vi "Exp03_GetGyroAngle.vi"() -> ()   [LabVIEW 2019]
uses:
  <vilib>/myRIO/Instrument Drivers/Onboard IO/I2C/typedefs/I2C User Configuration.ctl
  <vilib>/myRIO/Instrument Drivers/Onboard IO/I2C/typedefs/I2C Transfer Rate.ctl
  <vilib>/Platform/TimedLoop/XDataNode/timing_clust.ctl
  <vilib>/Platform/TimedLoop/XDataNode/nitl_modes.ctl
  <vilib>/Platform/TimedLoop/XDataNode/wakeup.ctl
  <vilib>/Utility/error.llb/Error Cluster From Error Code.vi
  <vilib>/myRIO/Common/Instrument Driver Framework/myRIO v1.0/I2C/vis/myRIO v1.0 Configure I2C.vi
  <vilib>/myRIO/Common/Instrument Driver Framework/myRIO v1.0/I2C/vis/myRIO v1.0 Write I2C.vi
  <vilib>/myRIO/Common/Instrument Driver Framework/myRIO v1.0/I2C/vis/myRIO v1.0 Read I2C.vi
  <vilib>/Platform/TimedLoop/XDataNode/XDataNode.xnode
  <vilib>/myRIO/Instrument Drivers/Onboard IO/I2C/I2C.lvlib
  <vilib>/Platform/TimedLoop/XDataNode/XDNodeRunTimeDep.lvlib
panel:
  out "gyro angle":dbl
  in  "zero":bool
  in  "initial bias":i16
  out "angular velocity":dbl
  out "acc angle":dbl
  out "Bytes Read (decimal)":u8[](array[numeric]) format="%0d"
  out "Gyro Z":i16
  out "Gyro X":i16
  out "Gyro Y":i16
  out "Acc Z":i16
  out "Temperature":dbl
  out "Acc Y":i16
  out "Acc X":i16
  in  "stop":bool
  out "error out":errorcluster
  out "Bytes Read (binary)":u8[](array[numeric]) format="%08b"
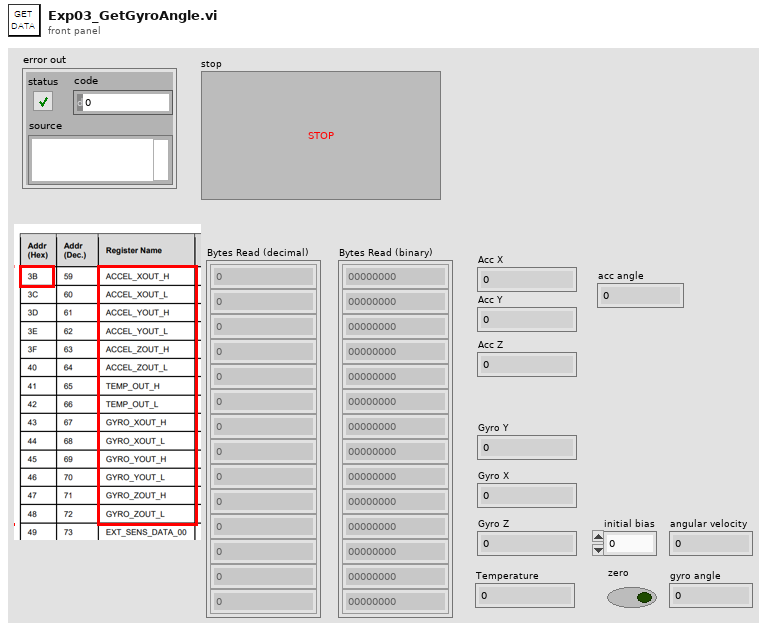
[diagram p1: front panel]
types:
  T1 = typedef "I2C.lvlib/I2C User Configuration.ctl" = cluster{"I2C Transfer Rate":T2}
  T2 = typedef "I2C.lvlib/I2C Transfer Rate.ctl" = enum16{"Standard mode (100 kbps)", "Fast mode (400 kbps)"}
  T3 = typedef "I2C.lvlib/I2C Reference.ctl" = cluster{"myRIO Reference":T4, "I2C Channels Enum":T8, "I2C Configuration":T9}
  T4 = typedef "myRIO Generic Hardware Reference.ctl" = cluster{"myRIO Model":T5, "myRIO Hardware Reference":T6}
  T5 = typedef "Hardware Version Enum.ctl" = enum16{"Unknown", "myRIO-1900", "myRIO-1950", "roboRIO", "NI ELVIS RIO CM", "ELVIS III"}
  T6 = typedef "myRIO v1.0 Reference.ctl" = cluster{"Generic FPGA Reference":T7, "Allow multiple opens":bool}
  T7 = typedef "Generic FPGA Reference.ctl" = refnum<k20>
  T8 = typedef "I2C Channels Enum.ctl" = enum16{"Not Connected", "A/I2C", "B/I2C", "I2C/I2C"}
  T9 = typedef "I2C.lvlib/I2C Configuration.ctl" = cluster{"I2C Transfer Rate":T2}
  T10 = typedef "XDNodeRunTimeDep.lvlib/timing_clust.ctl" = cluster{"Expected End [f-1]":u64, "Actual End [f-1]":u64, "Finished Late? [f-1]":bool, "Expected End [i-1]":u64, "Actual End [i-1]":u64, "Finished Late? [i-1]":bool, "Expected Start [i]":u64, "Actual Start [i]":u64, "Expected Start [f]":u64, "Actual Start [f]":u64, "Source Name":string, "Structure Name":string, "Period":i64, "Deadline":i64, "Offset":i64, "Start":i64, "Priority":i32, "Timeout":i32, "Mode":T11, "Wakeup Reason":T12, "Error":errorcluster, "Source Type":string, "Secondary Source Type":string, "Global End Time":u64, "Global Start Time":u64, "Frame Duration":u64, "Iteration Duration":u64, "Assigned CPU":i32, "I/O Scan Engine Mode":u32}
  T11 = typedef "XDNodeRunTimeDep.lvlib/nitl_modes.ctl" = enum32{"No Change", "Process missed periods, maintain original phase", "Discard missed periods, maintain original phase", "Process missed periods, ignore original phase", "Discard missed periods, ignore original phase"}
  T12 = typedef "XDNodeRunTimeDep.lvlib/wakeup.ctl" = enum32{"Normal", "Aborted", "Asynchronous wakeup", "Timing source error", "Timed loop error", "Timeout"}
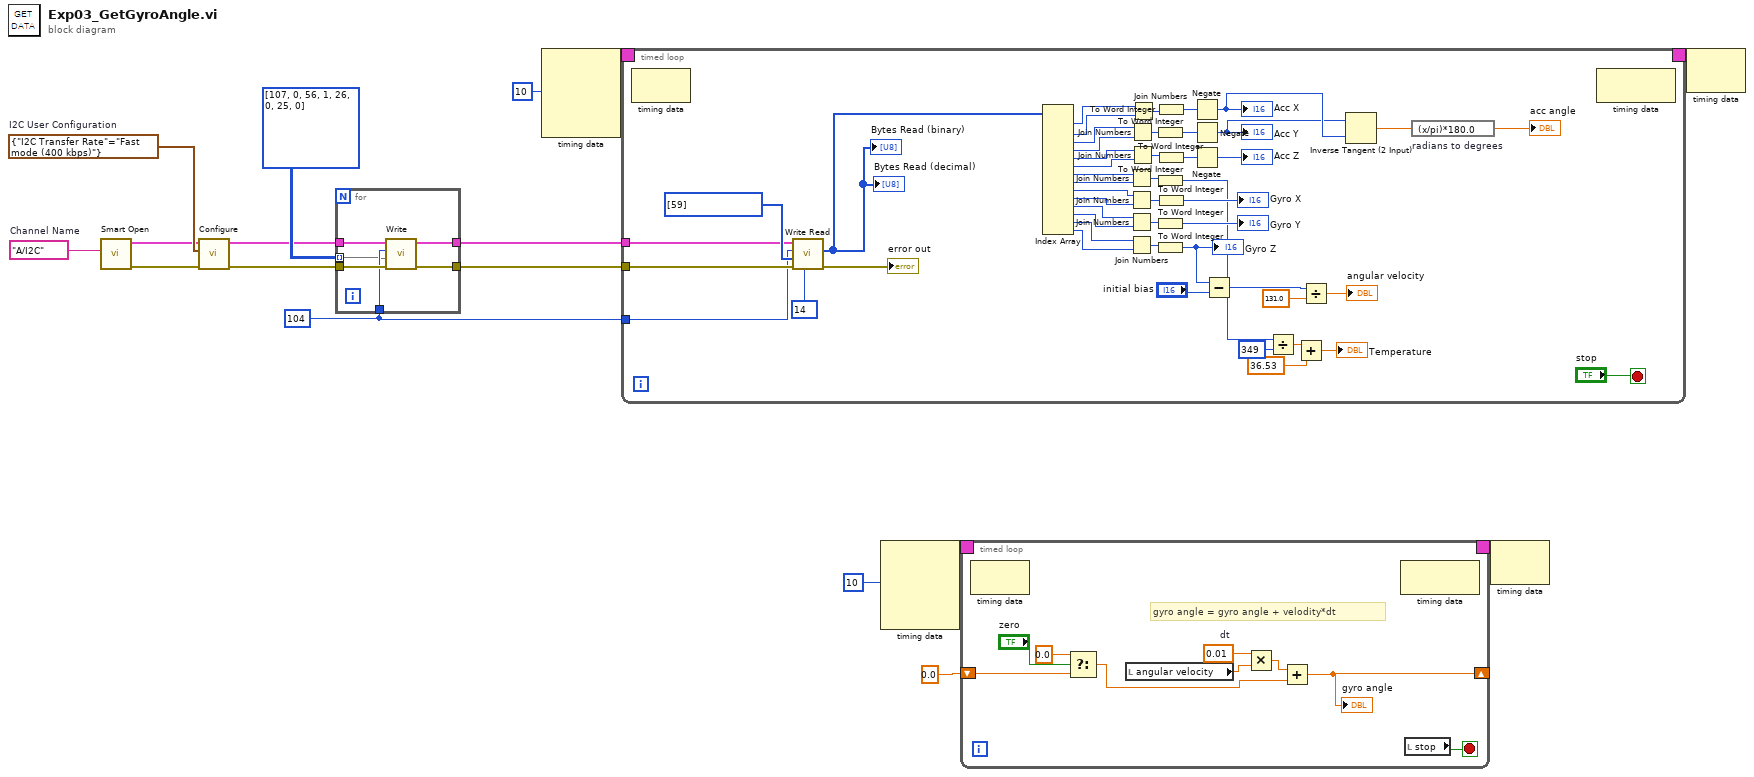
[diagram p0: block diagram]
diagram:
  w11 = u8 104 ("Slave Address (7-bit)")
  w16 = T1 {"I2C Transfer Rate"=enum."Fast mode (400 kbps)"}  # I2C User Configuration
  w17 = tag "A/I2C"  # Channel Name
  n1 = call <vilib>:"Smart Open.vi"("Channel Name"=w17) -> ("error out"=w14:errorcluster, "I2C Ref Out"=w15:T3)  [unwired: 9 in]
  n2 = call <vilib>:"Configure.vi"("error in (no error)"=w14, "I2C User Configuration"=w16, "I2C Ref In"=w15) -> ("error out"=w5:errorcluster, "I2C Ref Out"=w6:T3)  [unwired: 7 in]
  n3 = for {
    tunnel: w11 -> [w19]
    tunnel: w6 -> [w23]
    tunnel: [w20] -> w12
    tunnel: w5 -> [w22]
    tunnel: [w21] -> w13
    tunnel: u8[][] [[107, 0], [56, 1], [26, 0], [25, 0]] ("Bytes to Write") -> [w18] mode=indexing
    n4 = call <vilib>:"Write.vi"("error in (no error)"=w22, "Bytes to Write"=w18, "Slave Address (7-bit)"=w19, "I2C Ref In"=w23) -> ("error out"=w21:errorcluster, "I2C Ref Out"=w20:T3)  [unwired: 6 in]
  }
  n5 = node-c288(i64 10 ("Period")) -> (w10:T10)  [unwired: 3 in]
  n6 = timed-loop {
    timing: w10 -> [_]
    timing-out: [_] -> w9
    tunnel: w13 -> [w69]
    tunnel: w12 -> [w68]
    tunnel: w11 -> [w67]
    stop <- "stop" stop-if-true
    n7 = node-c288() -> ()  [unwired: 1 in, 1 out]
    n8 = call <vilib>:"Write Read.vi"("Byte Count"=u32 14, "error in (no error)"=w69, "Bytes to Write"=u8[] [59], "Slave Address (7-bit)"=w67, "I2C Ref In"=w68) -> ("error out"=→"error out":errorcluster, "Bytes Read"=w37:u8[])  [unwired: 3 in, 1 out]
    "Bytes Read (binary)" <- w37
    "Bytes Read (decimal)" <- w37
    n9 = Index Array(array=w37) -> (element #1=w65:u8, element #2=w64:u8, element #3=w63:u8, element #4=w62:u8, element #5=w61:u8, element #6=w60:u8, element #7=w59:u8, element #8=w58:u8, element #9=w57:u8, element #10=w56:u8, element #11=w55:u8, element #12=w54:u8, element #13=w53:u8, element #14=w52:u8)  [unwired: 14 in]
    n10 = Join Numbers(hi=w59, lo=w58) -> ((hi.lo)=w48:u16)
    n11 = Join Numbers(hi=w57, lo=w56) -> ((hi.lo)=w47:u16)
    n12 = Join Numbers(hi=w55, lo=w54) -> ((hi.lo)=w46:u16)
    n13 = Join Numbers(hi=w53, lo=w52) -> ((hi.lo)=w45:u16)
    n14 = Join Numbers(hi=w63, lo=w62) -> ((hi.lo)=w50:u16)
    n15 = Join Numbers(hi=w61, lo=w60) -> ((hi.lo)=w49:u16)
    n16 = Join Numbers(hi=w65, lo=w64) -> ((hi.lo)=w51:u16)
    n17 = To Word Integer(number=w50) -> (16bit integer=w32:i16)
    n18 = To Word Integer(number=w48) -> (16bit integer=w42:i16)
    n19 = To Word Integer(number=w46) -> (16bit integer=→"Gyro Y":i16)
    n20 = To Word Integer(number=w45) -> (16bit integer=w26:i16)
    "Gyro Z" <- w26
    n21 = To Word Integer(number=w51) -> (16bit integer=w34:i16)
    n22 = To Word Integer(number=w49) -> (16bit integer=w31:i16)
    n23 = To Word Integer(number=w47) -> (16bit integer=→"Gyro X":i16)
    n24 = Negate(x=w34) -> (-x=w33:i16)
    "Acc X" <- w33
    n25 = Negate(x=w32) -> (-x=w29:i16)
    "Acc Y" <- w29
    n26 = Negate(x=w31) -> (-x=→"Acc Z":i16)
    n27 = Subtract(x=w26, y="initial bias") -> (x-y=w24:i16)
    n28 = Divide(x=w42, y=i16 349) -> (x/y=w40:dbl)
    n29 = Add(x=w40, y=36.53) -> (x+y=→"Temperature":dbl)
    n30 = Divide(x=w24, y=131.0) -> (x/y=→"angular velocity":dbl)
    n31 = Inverse Tangent (2 Input)(1:w33, 2:w29) -> (0:w36:dbl)
    n32 = expression code="(x/pi)*180.0" "radians to degrees"(w36) -> (→"acc angle":dbl)
    n33 = node-c288() -> ()  [unwired: 1 in, 1 out]
  }
  n34 = node-c288(i64 10 ("Period")) -> (w4:T10)  [unwired: 3 in]
  n35 = timed-loop {
    timing: w4 -> [_]
    timing-out: [_] -> w3
    shift-right: [w76] -> _
    shift-left: 0.0 -> [w78]
    stop <- w75 stop-if-true
    w82 = 0.01  # dt
    # "gyro angle = gyro angle + velodity*dt"
    n36 = node-c288() -> ()  [unwired: 1 in, 1 out]
    n37 = Select(t=0.0, s="zero", f=w78) -> (s? t:f=w77:dbl)
    n38 = local read "angular velocity"() -> (w83:dbl)
    n39 = Multiply(x=w82, y=w83) -> (x*y=w81:dbl)
    n40 = Add(x=w81, y=w77) -> (x+y=w76:dbl)
    "gyro angle" <- w76
    n41 = node-c288() -> ()  [unwired: 1 in, 1 out]
    n42 = local read "stop"() -> (w75:bool)
  }
  n43 = node-c288(w3) -> ()  [unwired: 1 out]
  n44 = node-c288(w9) -> ()  [unwired: 1 out]
